vi "Dig.vi"(4 "Hooks Search Path":path[](array[path]), 6 "Execute Hooks?":cluster{"Pre":bool, "Post":bool}={"Pre"=TRUE, "Post"=TRUE}, 8 "Error In":errorcluster, 10 "Selection List":refnum<vi>[](array[refnum]), 11 "VI In":refnum<vi>) -> (0 "Error Out":errorcluster, 2 "Change Made?":bool, 3 "VI Out":refnum<vi>)   [LabVIEW 2018, in "Toolkit.lvlib"]
doc: "Encloses the selected objects in a Diagram Disable Structure, adds a RIP bookmark tag with an ISO 8601 timestamp and user name in parentheses, creates a copy of the Disabled frame and uses the copy for the Enabled frame, adds a \"Corpse\" subdiagram label to the Disabled frame, and adds a \"Spirit\" subdiagram label to the Enabled frame. The result is a \"grave\" for refactoring the code."
uses:
  Toolkit.lvlib
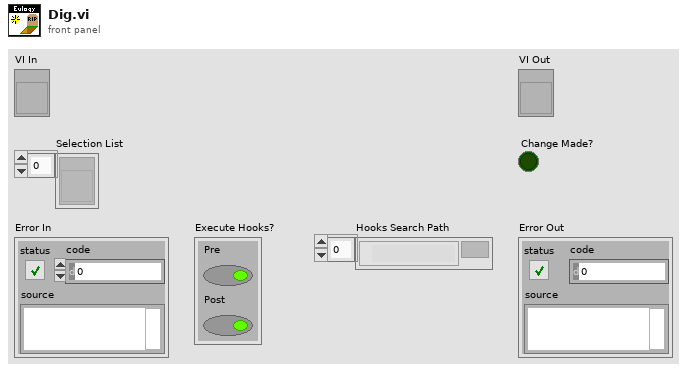
[diagram p1: front panel]
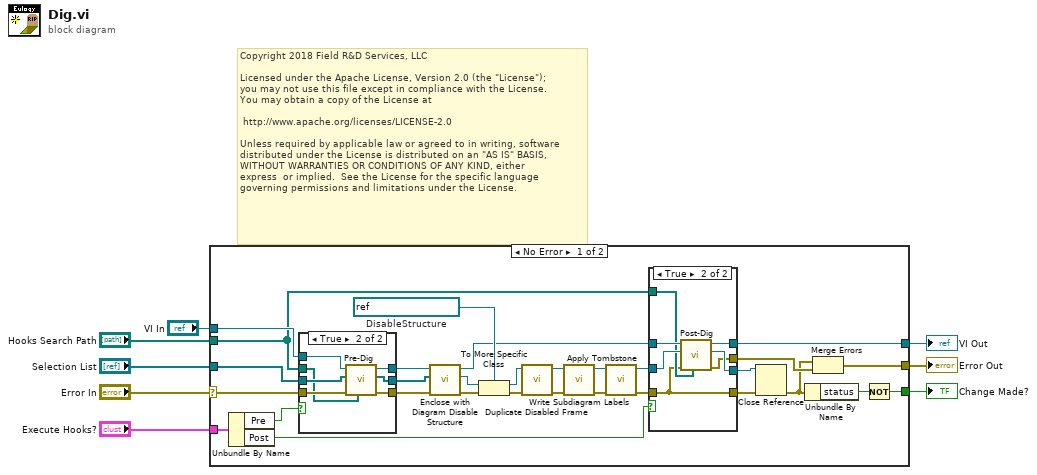
[diagram p0: block diagram]
diagram:
  # "Copyright 2018 Field R&D Services, LLC\n\nLicensed under the Apache License, Version 2.0 (the \"License\");\nyou may not use this file except in compliance with the License.\nYou may obtain a copy of the License at\n\n\thttp://www.apache.org/licenses/LICENSE-2.0\n\nUnless required by applicable law or agreed to in writing, software\ndistributed under the License is distributed on an \"AS IS\" BASIS,\nWITHOUT WARRANTIES OR CONDITIONS OF ANY KIND, either \nexpress  or implied.  See the License for the specific language \ngoverning permissions and limitations under the License."
  n1 = case shown="No Error" "Error In" {
    selector: "Error In" -> [w25 w59]
    tunnel: [w22 w60] -> w8
    tunnel: "VI In" -> [w29 w60]
    tunnel: "Selection List" -> [w24 _]
    tunnel: [w13 w59] -> w5
    tunnel: "Hooks Search Path" -> [w17 _]
    tunnel: "Execute Hooks?" -> [w16 _]
    tunnel: [w9 _] -> w1
    frame No Error {
      w37 = refnum<vi> refnum  # DisableStructure
      n2 = Unbundle By Name(w16) -> ("Pre"=w15:bool, "Post"=w14:bool)
      n3 = case shown="True" w15 {
        tunnel: w29 -> [w51 w58]
        tunnel: [w51 w57] -> w28
        tunnel: [w50 w56] -> w27
        tunnel: [w49 w55] -> w26
        tunnel: w25 -> [w49 w54]
        tunnel: w24 -> [w50 w53]
        tunnel: w17 -> [_ w52]
        frame False {
        }
        frame True {
          n4 = call "Pre-Dig.vi"("Search Path"=w52, "Error In"=w54, "Selection List[] In"=w53, "VI In"=w58) -> ("Error Out"=w55:errorcluster, "Selection List[] Out"=w56:refnum<vi>[], "VI Out"=w57:refnum<vi>)  [unwired: 5 in]
        }
      }
      n5 = call "Enclose with Diagram Disable Structure.vi"("Error In"=w26, "Selection List[]"=w27, "VI In"=w28) -> ("Error Out"=w31:errorcluster, "Structure"=w38:refnum<vi>, "VI Out"=w23:refnum<vi>)  [unwired: 6 in]
      n6 = To More Specific Class(target class=w37, reference=w38, error in=w31) -> (specific class reference=w36:refnum<vi>, error out=w35:errorcluster)
      n7 = call "Duplicate Disabled Frame.vi"("Error In"=w35, "DisableStructure In"=w36) -> ("Error Out"=w34:errorcluster, "DisableStructure Out"=w33:refnum<vi>)  [unwired: 8 in]
      n8 = call "Write Subdiagram Labels.vi"("Error In"=w34, "DisableStructure In"=w33) -> ("Error Out"=w30:errorcluster, "DisableStructure Out"=w32:refnum<vi>)  [unwired: 8 in]
      n9 = call "Apply Tombstone.vi"("Error In"=w30, "Grave In"=w32) -> ("Error Out"=w20:errorcluster, "Grave Out"=w21:refnum<vi>)  [unwired: 8 in]
      n10 = case shown="True" w14 {
        tunnel: w23 -> [w41 w48]
        tunnel: [w41 w47] -> w22
        tunnel: w21 -> [w40 w46]
        tunnel: w20 -> [w39 w42]
        tunnel: [w39 w42] -> w19
        tunnel: [w40 w45] -> w18
        tunnel: w17 -> [_ w44]
        tunnel: [_ w43] -> w12
        frame False {
        }
        frame True {
          n11 = call "Post-Dig.vi"("Search Path"=w44, "Error In"=w42, "Grave In"=w46, "VI In"=w48) -> ("Error Out"=w43:errorcluster, "Grave Out"=w45:refnum<vi>, "VI Out"=w47:refnum<vi>)  [unwired: 5 in]
        }
      }
      n12 = Close Reference(reference=w18, error in (no error)=w19) -> (error out=w11:errorcluster)
      n13 = Unbundle By Name(w11) -> ("status"=w10:bool)
      n14 = Merge Errors(w11, w12) -> (w13:errorcluster)
      n15 = Not(x=w10) -> (.not. x?=w9:bool)
    }
    frame Error {
    }
  }
  "Error Out" <- w5
  "VI Out" <- w8
  "Change Made?" <- w1
